vi "WS1050 CAPDAC Setting.vi"(6 "DUT Mask Mode (All)":T1=enum."All", 8 "error in":errorcluster, 9 "C3 Cap DAC":u8=128 caption="B Data In" format="0x%02x", 10 "C2 Cap DAC":u8=128 caption="B Data In" format="0x%02x", 11 "C1 Cap DAC":u8=128 caption="B Data In" format="0x%02x") -> (0 "error out":errorcluster)   [LabVIEW 2012]
uses:
  WS_VCAP Driver 029/Source/WSVCAP Shell/Type Defs/WSVCAP SHL I2C DUT Mask Mode Enum.ctl
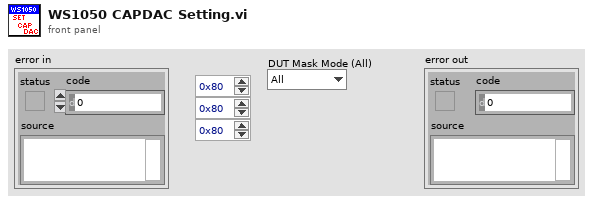
[diagram p1: front panel]
types:
  T1 = typedef "WSVCAP SHL I2C DUT Mask Mode Enum.ctl" = enum16{"Custom", "C1", "C2", "C3", "All"}
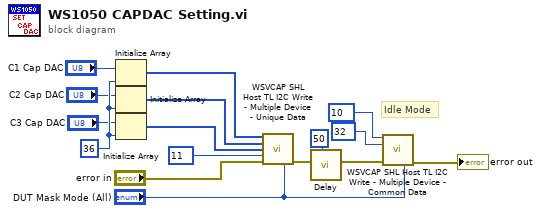
[diagram p0: block diagram]
diagram:
  w16 = 36 ("dimension size")
  # "Idle Mode"
  n1 = Initialize Array("C1 Cap DAC", w16) -> (w8:u8[])
  n2 = Initialize Array("C2 Cap DAC", w16) -> (w7:u8[])
  n3 = Initialize Array("C3 Cap DAC", w16) -> (w6:u8[])
  n4 = call "WSVCAP SHL Host TL I2C Write - Multiple Device - Unique Data.vi"("C1 Data"=w8, "C2 Data"=w7, "C3 Data"=w6, "Sub Address"=u8 11, "error in"="error in", "DUT Mask Mode (All)"="DUT Mask Mode (All)") -> ("error out"=w10:errorcluster)  [unwired: 9 in]
  n5 = call "Delay.vi"("milliseconds to wait"=u32 50, "error in (no error)"=w10) -> ("error out"=w2:errorcluster)  [unwired: 9 in]
  n6 = call "WSVCAP SHL Host TL I2C Write - Multiple Device - Common Data.vi"("Sub Address"=u8 10, "Data Out [U8]"=u8 32 ("Sub Address"), "error in"=w2, "DUT Mask Mode (All)"="DUT Mask Mode (All)") -> ("error out"=→"error out":errorcluster)  [unwired: 11 in]
